vi "Write Key.vi"(8 "error in":errorcluster, 9 "Value":string, 10 "Key":string, 11 "E2E configuration in":refnum<class "E2E Tag Exchange configuration.lvclass">) -> (0 "error out":errorcluster, 3 "E2E configuration out":refnum<class "E2E Tag Exchange configuration.lvclass">)   [LabVIEW 2015, in "E2E Tag Exchange configuration.lvclass"]
uses:
  E2E Tag Exchange configuration.lvclass
  E2E Tag Exchange configuration.lvclass/E2E Tag Exchange configuration.ctl
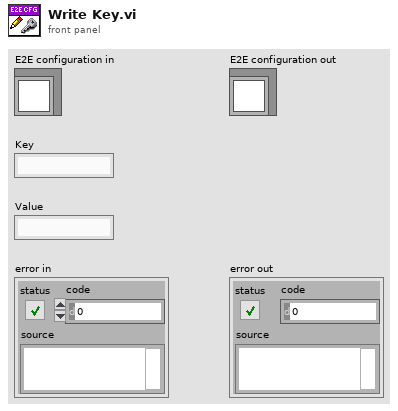
[diagram p1: front panel]
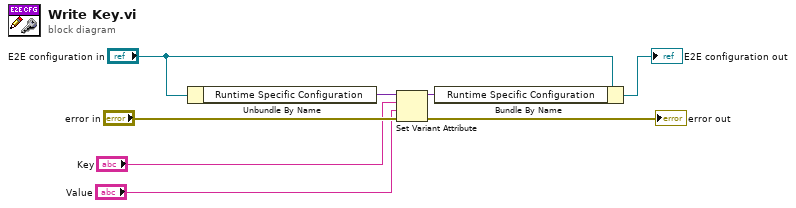
[diagram p0: block diagram]
diagram:
  n1 = Unbundle By Name("E2E configuration in") -> ("Runtime Specific Configuration"=w8:variant)
  n2 = Set Variant Attribute(Variant=w8, name="Key", value="Value", error in="error in") -> (Variant out=w6:variant, error out=→"error out":errorcluster)  [unwired: 1 out]
  n3 = Bundle By Name(cluster="E2E configuration in", "Runtime Specific Configuration"=w6) -> (→"E2E configuration out":refnum<class "E2E Tag Exchange configuration.lvclass">)
